vi "File.ArchiveMover, Assign Task.vi"(6 "SubDirs":string[](array[string]), 7 "Q Name":string="FileMover", 8 "error in":errorcluster, 9 "New Name":string, 10 "DestDir":path, 11 "Source":path) -> (0 "error out":errorcluster)   [LabVIEW 2018]
uses:
  File.ArchiveMover Task.ctl
  <vilib>/KATE/Queues/Queue Utils.lvlib
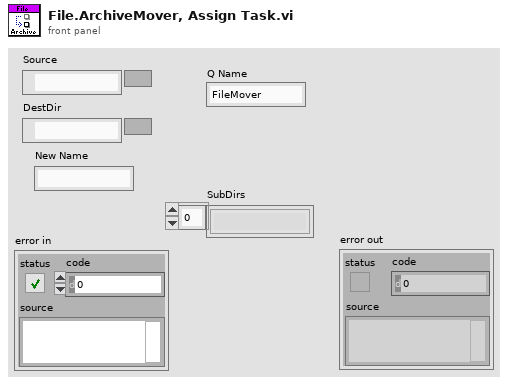
[diagram p1: front panel]
types:
  T1 = typedef "File.ArchiveMover Task.ctl" = cluster{"Source":path, "DestDir":path, "New Name":string, "SubDirs":string[]}
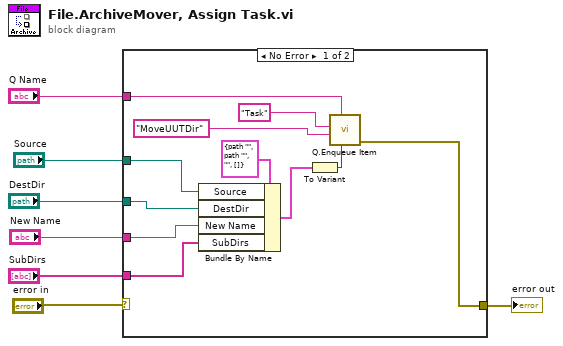
[diagram p0: block diagram]
diagram:
  n1 = case shown="No Error" "error in" {
    selector: "error in" -> [_ w19]
    tunnel: "Q Name" -> [w18 _]
    tunnel: "Source" -> [w13 _]
    tunnel: "DestDir" -> [w12 _]
    tunnel: [w16 w19] -> w4
    tunnel: "SubDirs" -> [w10 _]
    tunnel: "New Name" -> [w11 _]
    frame No Error {
      n2 = Bundle By Name(cluster=T1 {"Source"=path "", "DestDir"=path "", "New Name"="", "SubDirs"=[]} ("output cluster"), "Source"=w13, "DestDir"=w12, "New Name"=w11, "SubDirs"=w10) -> (w8:T1)
      n3 = To Variant(anything=w8) -> (Variant=w17:variant)
      n4 = call <vilib>:"Q.Enqueue Item.vi"("Data1"=w17, "Q Name"=w18, "Sub"="MoveUUTDir" ("Task Name"), "Cmd"="Task" ("Task Name")) -> ("error out"=w16:errorcluster)  [unwired: 6 in, 1 out]
    }
    frame Error {
    }
  }
  "error out" <- w4
